vi "EXDIR-YAML_IsFloatingColon.vi"(11 "String":string) -> (3 "after the 1st char is empty or all spaces":bool)   [LabVIEW 2016]
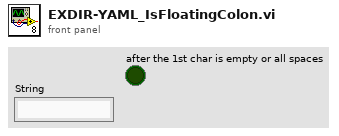
[diagram p1: front panel]
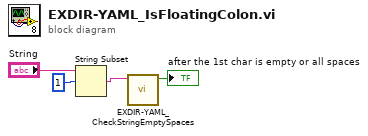
[diagram p0: block diagram]
diagram:
  n1 = String Subset(string="String", offset (0)=1) -> (substring=w2:string)  [unwired: 1 in]
  n2 = call "EXDIR-YAML_CheckStringEmptySpaces.vi"("String"=w2) -> ("empty or all spaces"=→"after the 1st char is empty or all spaces":bool)  [unwired: 10 in]
